vi "Scaled Window for 1 Chan.vi"(8 "error in (no error)":errorcluster, 9 "window parameter":dbl=nan, 10 "window":T1 items=["Rectangle"=0, "Hanning"=1, "Hamming"=2, "Blackman-Harris"=3, "Exact Blackman"=4, "Blackman"=5, "Flat Top"=6, "4 Term B-Harris "=7, "7 Term B-Harris"=8, "Low Sidelobe"=9, "Blackman Nuttall"=11, "Triangle"=30, "Bartlett-Hanning"=31, "Bohman"=32, "Parzen"=33, "Welch"=34, "Kaiser"=60, "Dolph-Chebyshev"=61, "Gaussian"=62], 11 "signal in":waveform(dbl)) -> (0 "error out":errorcluster, 2 "window constants":cluster{"eq noise BW":dbl, "coherent gain":dbl} {"coherent gain" format="%.6f"; "eq noise BW" format="%.6f"}, 3 "signal out":waveform(dbl))   [LabVIEW 2020, in "NI_MAPro.lvlib"]
doc: "Applies a scaled window to the time-domain signal and outputs window constants for further analysis. Wire data to the <B>signal in</B> input to determine the polymorphic instance to use or manually select the instance."
uses:
  NI_MAPro.lvlib
  windowTd.ctl
  NI_MABase.lvlib
  NI_AALPro.lvlib
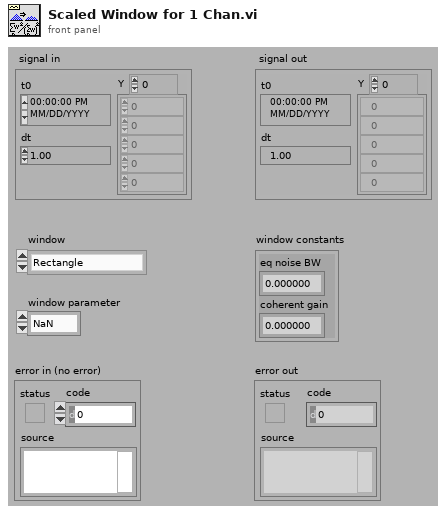
[diagram p1: front panel]
types:
  T1 = typedef "NI_AALPro.lvlib/windowTd.ctl" = u32
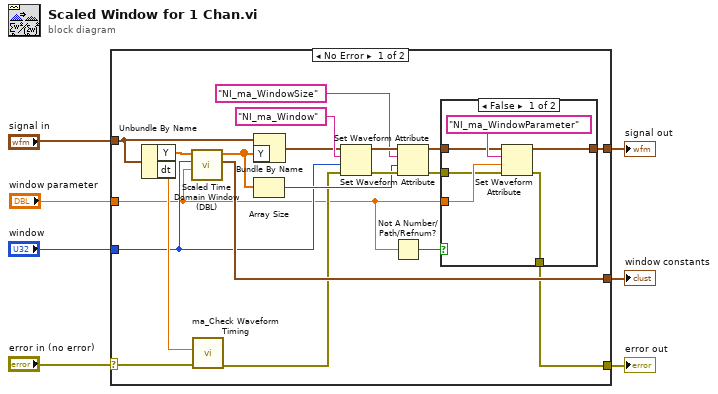
[diagram p0: block diagram]
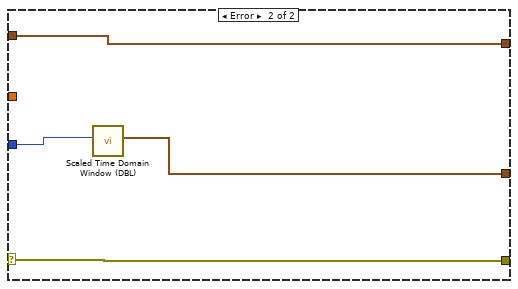
[diagram p3: hidden frame]
diagram:
  n1 = case shown="No Error" "error in (no error)" {
    selector: "error in (no error)" -> [w24 w36]
    tunnel: "window" -> [w16 w37]
    tunnel: [w27 w38] -> w7
    tunnel: [w14 w39] -> w5
    tunnel: "signal in" -> [w26 w39]
    tunnel: [w13 w36] -> w2
    tunnel: "window parameter" -> [w8 _]
    frame No Error {
      n2 = Unbundle By Name(w26) -> ("Y"=w25:dbl[], "dt"=w23:dbl)
      n3 = call "Scaled Time Domain Window (DBL).vi"("window parameter"=w8, "window"=w16, "X"=w25) -> ("window properties"=w27:cluster{"eq noise BW":dbl, "coherent gain":dbl}, "Windowed X"=w11:dbl[])  [unwired: 6 in, 1 out]
      n4 = call "ma_Check Waveform Timing.vi"("error in (no error)"=w24, "dt"=w23) -> ("error out"=w10:errorcluster)  [unwired: 8 in, 1 out]
      n5 = Bundle By Name(cluster=w26, "Y"=w11) -> (w19:waveform(dbl))
      n6 = Array Size(array=w11) -> (size(s)=w17:i32)
      n7 = Set Waveform Attribute(4:w10, 5:w16, 6:"NI_ma_Window" ("name"), 7:w19) -> (0:w18:errorcluster, 3:w22:waveform(dbl))  [unwired: 1 out]
      n8 = Not A Number/Path/Refnum?(number/path/refnum=w8) -> (NaN/Path/Refnum?=w9:bool)
      n9 = Set Waveform Attribute(4:w18, 5:w17, 6:"NI_ma_WindowSize" ("name"), 7:w22) -> (0:w12:errorcluster, 3:w15:waveform(dbl))  [unwired: 1 out]
      n10 = case shown="False" w9 {
        tunnel: w15 -> [w32 w35]
        tunnel: [w31 w35] -> w14
        tunnel: w8 -> [w30 _]
        tunnel: [w29 w34] -> w13
        tunnel: w12 -> [w28 w34]
        frame False {
          n11 = Set Waveform Attribute(4:w28, 5:w30, 6:"NI_ma_WindowParameter" ("name"), 7:w32) -> (0:w29:errorcluster, 3:w31:waveform(dbl))  [unwired: 1 out]
        }
        frame True {
        }
      }
    }
    frame Error {
      n12 = call "Scaled Time Domain Window (DBL).vi"("window"=w37) -> ("window properties"=w38:cluster{"eq noise BW":dbl, "coherent gain":dbl})  [unwired: 8 in, 2 out]
    }
  }
  "window constants" <- w7
  "error out" <- w2
  "signal out" <- w5
